vi "RubikStart.vi"() -> ()   [LabVIEW 2017]
uses:
  Projekt-RubikLibrary/ServoEnumControl.ctl
  Projekt-RubikLibrary/ServoAbsAngleControl.ctl
  Projekt-RubikLibrary/RubikLibrary.lvlib
panel:
  in  "List of Servo Angles":T1[](array[typedef])
  in  "Gripper closed":bool=TRUE
  in  "List of Servos":T2[](array[typedef])=[enum."Left Servo", enum."Front Servo", enum."Right Servo"]
  # "Rubic Start"
  # "Rubik Cube Start Configuration\n\nPosition of Grippers:  Open\nPosition of Servos: -90°"
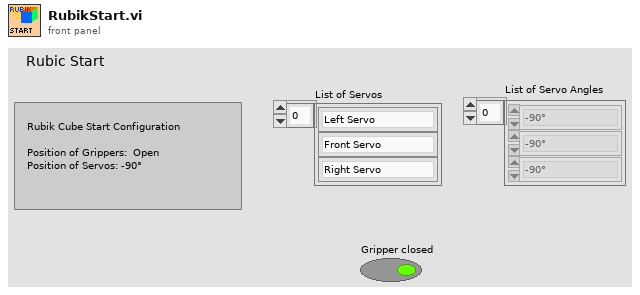
[diagram p1: front panel]
types:
  T1 = typedef "RubikLibrary.lvlib/ServoAbsAngleControl.ctl" = enum16{"+90°", "0°", "-90°"}
  T2 = typedef "RubikLibrary.lvlib/ServoEnumControl.ctl" = enum16{"Left Servo", "Front Servo", "Right Servo"}
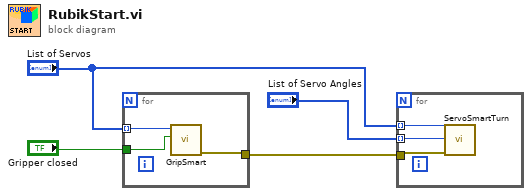
[diagram p0: block diagram]
diagram:
  n1 = for {
    tunnel: "List of Servos" -> [w7] mode=indexing
    tunnel: "Gripper closed" -> [w6]
    tunnel: [w5] -> w2
    n2 = call "GripSmart.vi"("Grip closed (in)"=w6, "Servo"=w7) -> ("error out"=w5:errorcluster)  [unwired: 8 in, 1 out]
  }
  n3 = for {
    tunnel: "List of Servos" -> [w10] mode=indexing
    tunnel: w2 -> [w9]
    tunnel: "List of Servo Angles" -> [w8] mode=indexing
    n4 = call "ServoSmartTurn.vi"("error in"=w9, "Turn to (in)"=w8, "Servo"=w10) -> ()  [unwired: 7 in, 2 out]
  }
